vi "grSim Packet Command.vi"(5 "BallRef":refnum<class "Ball.lvclass">, 6 "repalceBall":bool, 7 "ReplaceRobots":bool, 8 "grSIM replacement":T1, 9 "FIRASim?":bool=TRUE, 10 "Robots":T4[](array[typedef]), 11 "isteamyellow":bool=TRUE) -> (1 "Array":u8[](array[numeric]))   [LabVIEW 2020]
uses:
  Convert AI Robot to Robot Command Folder/grSim/grSim Robot Command.ctl
  Ball_class/Ball.lvclass
  Controls/grSimReplacement.ctl
  grSim RobotReplacement.ctl
  grSim_BallReplacement.ctl
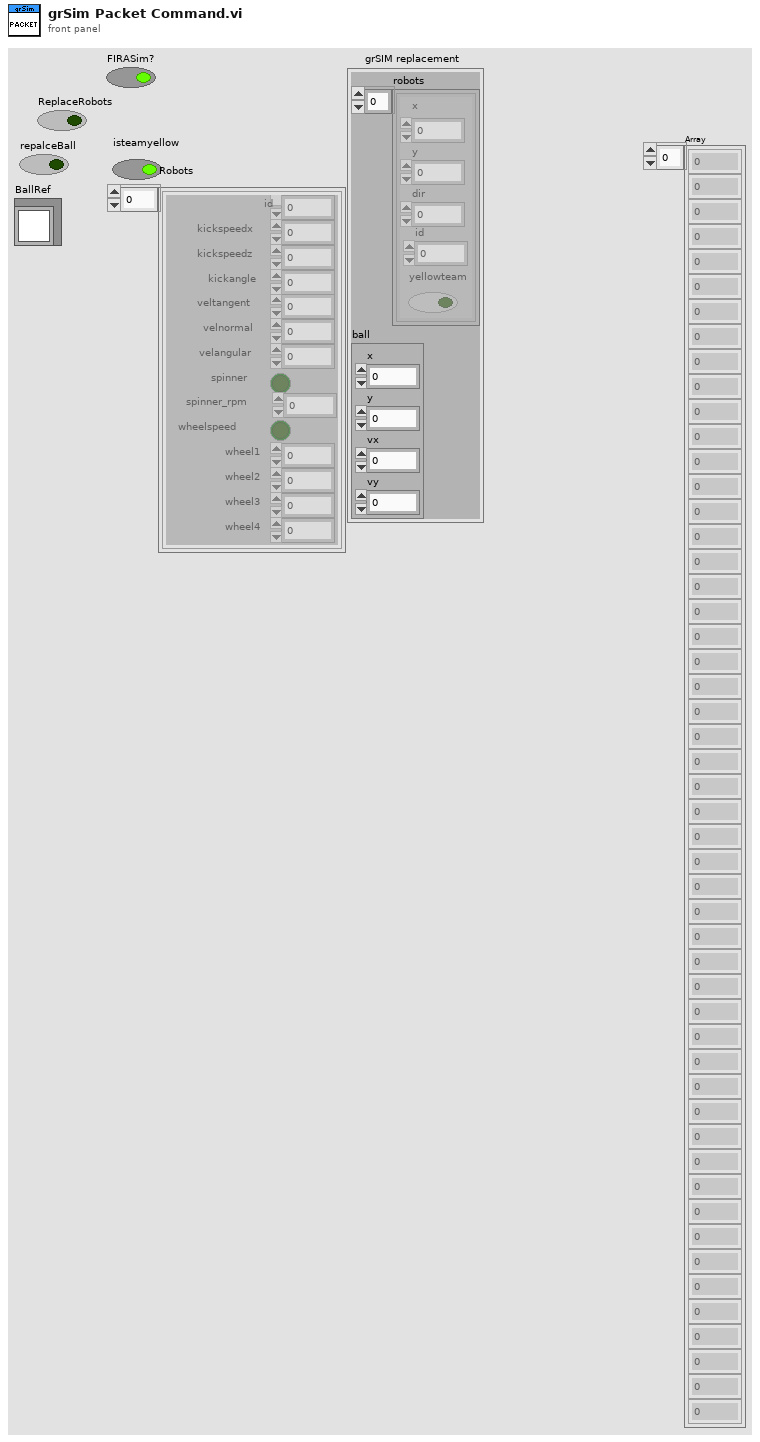
[diagram p1: front panel]
types:
  T1 = typedef "grSimReplacement.ctl" = cluster{"robots":T2[], "ball":T3}
  T2 = typedef "grSim RobotReplacement.ctl" = cluster{"x":dbl, "y":dbl, "dir":dbl, "yellowteam":bool, "id":u32}
  T3 = typedef "grSim_BallReplacement.ctl" = cluster{"x":dbl, "y":dbl, "vx":dbl, "vy":dbl}
  T4 = typedef "grSim Robot Command.ctl" = cluster{"id":u32, "kickspeedx":sgl, "kickspeedz":sgl, "veltangent":sgl, "velnormal":sgl, "velangular":sgl, "spinner":bool, "wheelspeed":bool, "wheel1":sgl, "wheel2":sgl, "wheel3":sgl, "wheel4":sgl, "kickangle":sgl, "spinner_rpm":sgl}
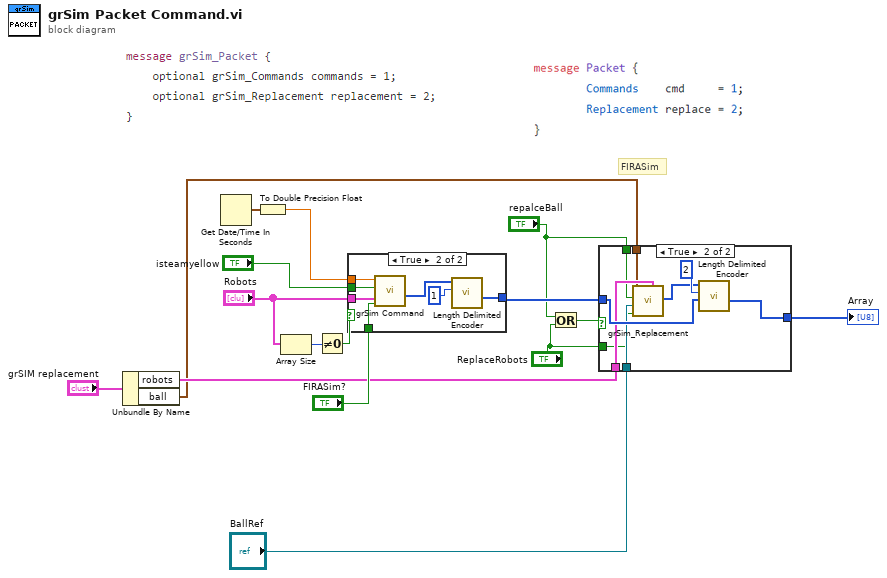
[diagram p0: block diagram]
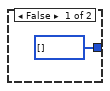
[diagram p3: hidden frame]
diagram:
  # "FIRASim"
  n1 = Unbundle By Name("grSIM replacement") -> ("robots"=w2:T2[], "ball"=w1:T3)
  n2 = Get Date/Time In Seconds() -> (seconds since 1Jan1904=w15:timestamp)
  n3 = To Double Precision Float(number=w15) -> (double precision float=w14:dbl)
  n4 = Array Size(array="Robots") -> (size(s)=w12:i32)
  n5 = Not Equal To 0?(x=w12) -> (x != 0?=w11:bool)
  n6 = case shown="True" w11 {
    tunnel: "isteamyellow" -> [_ w22]
    tunnel: w14 -> [_ w21]
    tunnel: [u8[] [] ("Array") w20] -> w9
    tunnel: "Robots" -> [_ w19]
    tunnel: "FIRASim?" -> [_ w18]
    frame False {
    }
    frame True {
      n7 = call "grSim Command.vi"("FIRASim?"=w18, "Robots"=w19, "isteamyellow"=w22, "timestamp"=w21) -> ("Command"=w24:u8[])  [unwired: 7 in]
      n8 = call "Length Delimited Encoder.vi"("Key"=u32 1, "Array In to be added"=w24) -> ("Array"=w20:u8[])  [unwired: 9 in]
    }
  }
  n9 = Or(x="repalceBall", y="ReplaceRobots") -> (x .or. y?=w6:bool)
  n10 = case shown="True" w6 {
    tunnel: [w25 w34] -> w10
    tunnel: w9 -> [w25 w33]
    tunnel: w2 -> [_ w32]
    tunnel: "repalceBall" -> [_ w31]
    tunnel: "BallRef" -> [_ w30]
    tunnel: "ReplaceRobots" -> [_ w27]
    tunnel: w1 -> [_ w26]
    frame False {
    }
    frame True {
      n11 = call "grSim_Replacement.vi"("grSim_RobotReplacement"=w32, "ReplaceRobots"=w27, "BallRef"=w30, "repalceBall"=w31, "grSim_BallReplacement"=w26) -> ("Array"=w28:u8[])  [unwired: 6 in]
      n12 = call "Length Delimited Encoder.vi"("Original Array In"=w33, "Key"=u32 2, "Array In to be added"=w28) -> ("Array"=w34:u8[])  [unwired: 8 in]
    }
  }
  "Array" <- w10
